vi "avaliaBolaDentroArea.vi"(10 "balls":T1[](array[typedef]), 11 "IA State":T2={"our_robots"=[], "enemy_robots"=[], "balls"=[], "geometry"={"field_length"=0, "field_width"=0, "goal_width"=0, "goal_depth"=0, "center_circle_radius"=0, "defense_width"=0, "defense_depth"=0, "free_kick_from_defense_dist"=0, "penalty_spot_from_field_line_dist"=0, "penalty_line_from_spot_dist"=0, "half_moon_depth"=0, "half_moon_width"=0}, "IA Judge"={"stage"="", "command"="", "our_goalie_id"=0.0, "enemy_goalie_id"=0.0, "command enum"=enum."Halt", "Time"=enum."Azul"}, "Received Timestamp"=timestamp(0 s since 1904-01-01), "Events"={"Touch"=FALSE, "id touch"=0.0, "Ball out of \nVision"=FALSE, "Ball inside \nGoalie area"=FALSE, "Robot not responding"=FALSE, "Robots responding status"=[1.0, 1.0, 1.0, 1.0, 1.0, 1.0], "Enemy Ball \nPossession"=FALSE, "Id ini Possession"=0.0, "Ball Possesion"=FALSE, "Id Possesion"=0.0, "Ball at\nour goal side"=FALSE, "Ball at\ntouchline"=FALSE, "Ball at\nenemy goal side"=FALSE}}) -> (3 "Bola dentro da área":bool=TRUE)   [LabVIEW 2018]
uses:
  2019/VSS/Core/AI Input.ctl
  2019/VSS/Core/AI Robot.ctl
  2019/VSS/Intel/Functions Enum.ctl
  2019/VSS/Intel/AttackerStates.ctl
  2019/VSS/Path Planning/RRT/PathDests.ctl
  2019/VSS/Path Planning/RRT/PathDest.ctl
  2019/VSS/Core/AI Ball.ctl
  2019/VSS/Core/Field Size.ctl
  2019/VSS/Core/AI Judge.ctl
  2019/VSS/Intel/Command Enum.ctl
  2019/VSS/Util/Events/Events.ctl
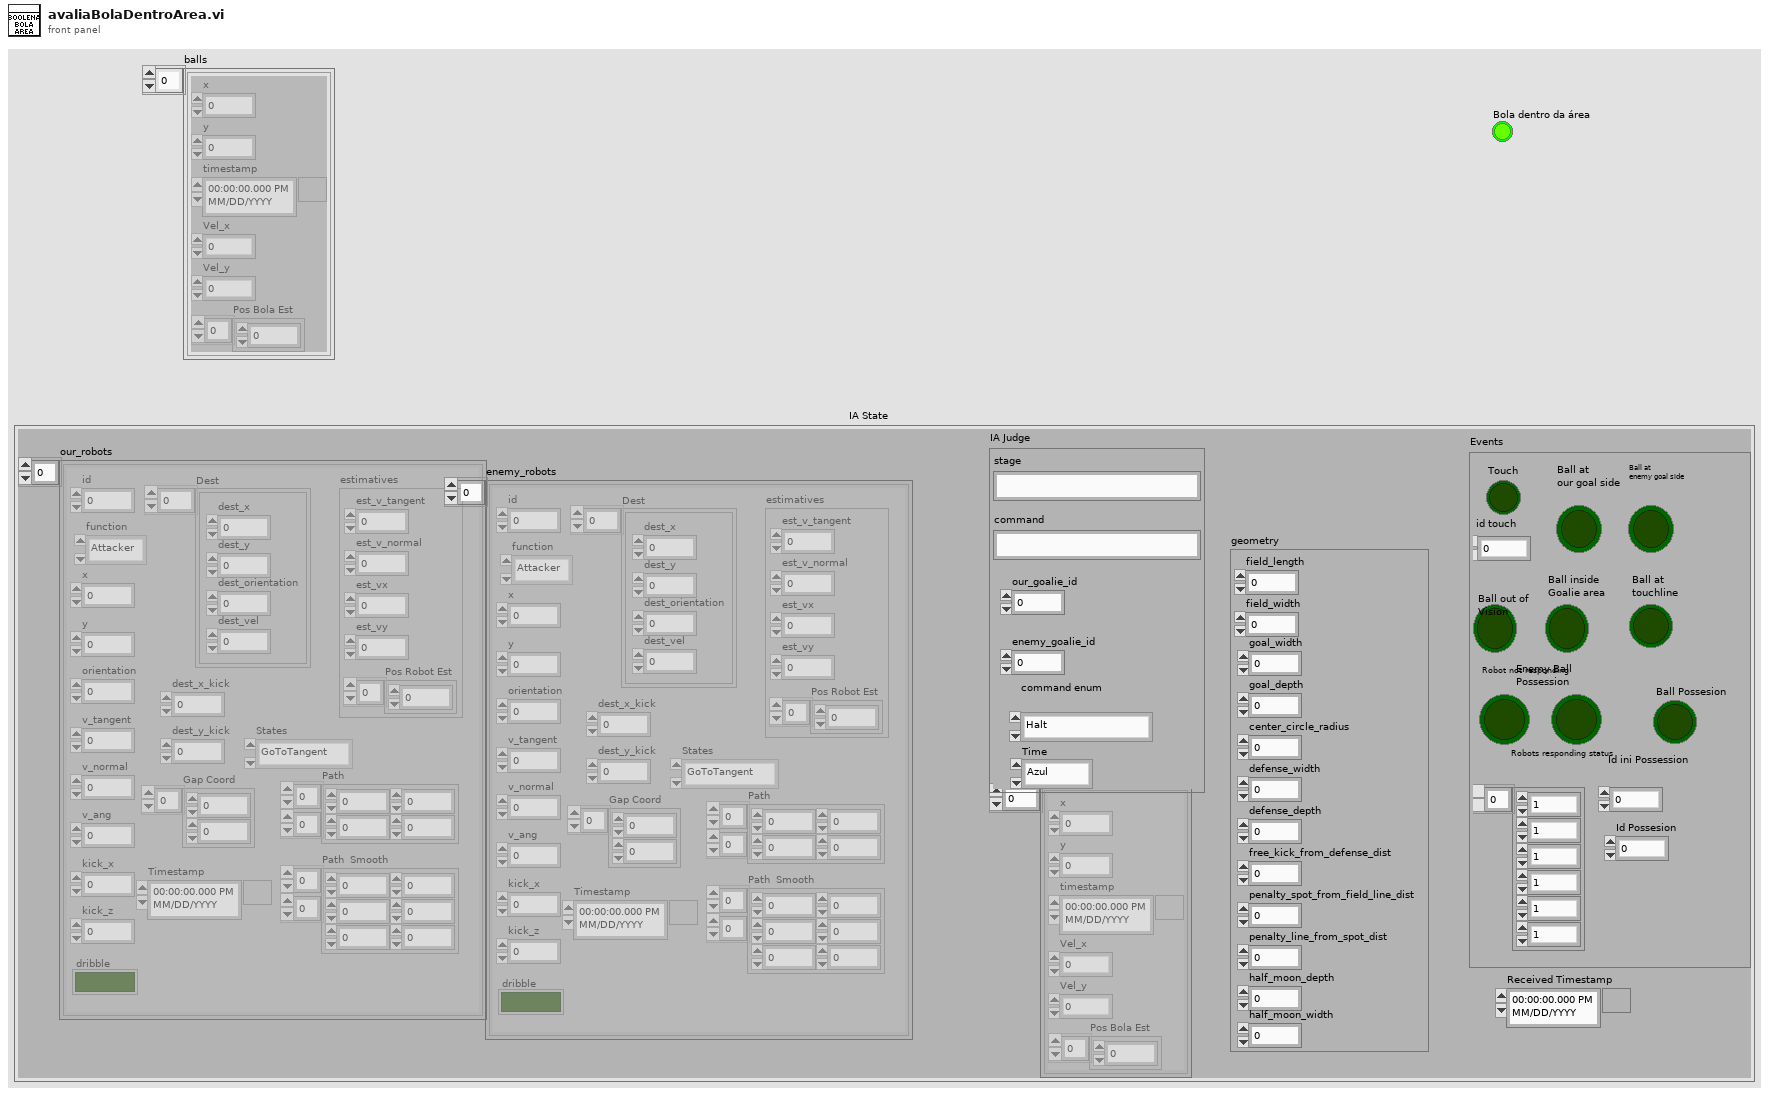
[diagram p1: front panel]
types:
  T1 = typedef "AI Ball.ctl" = cluster{"x":dbl, "y":dbl, "timestamp":timestamp, "Vel_x":dbl, "Vel_y":dbl, "Pos Bola Est":dbl[]}
  T2 = typedef "AI Input.ctl" = cluster{"our_robots":T3[], "enemy_robots":T3[], "balls":T1[], "geometry":T8, "IA Judge":T9, "Received Timestamp":timestamp, "Events":T11}
  T3 = typedef "AI Robot.ctl" = cluster{"id":u32, "function":T4, "x":dbl, "y":dbl, "orientation":dbl, "v_tangent":dbl, "v_normal":dbl, "v_ang":dbl, "kick_x":dbl, "kick_z":dbl, "dribble":bool, "Timestamp":timestamp, "estimatives":cluster{"est_v_tangent":dbl, "est_v_normal":dbl, "est_vx":dbl, "est_vy":dbl, "Pos Robot Est":dbl[]}, "dest_x_kick":dbl, "dest_y_kick":dbl, "Gap Coord":dbl[], "States":T5, "Path ":dbl[][], "Path  Smooth":dbl[][], "Dest":T6}
  T4 = typedef "Functions Enum.ctl" = enum16{"Attacker", "Goalie", "Defender", "Striker", "Goto 0", "Dummy", "Kicker", "ZigZag"}
  T5 = typedef "AttackerStates.ctl" = enum16{"Pass", "GoToTangent", "BallGetting", "GoToKick", "Rotate anti-clockwise", "Rotate Clockwise", ""}
  T6 = typedef "PathDests.ctl" = T7[]
  T7 = typedef "PathDest.ctl" = cluster{"dest_x":dbl, "dest_y":dbl, "dest_orientation":dbl, "dest_vel":dbl}
  T8 = typedef "Field Size.ctl" = cluster{"field_length":u32, "field_width":u32, "goal_width":u32, "goal_depth":u32, "center_circle_radius":u32, "defense_width":u32, "defense_depth":u32, "free_kick_from_defense_dist":u32, "penalty_spot_from_field_line_dist":u32, "penalty_line_from_spot_dist":u32, "half_moon_depth":u32, "half_moon_width":u32}
  T9 = typedef "AI Judge.ctl" = cluster{"stage":string, "command":string, "our_goalie_id":dbl, "enemy_goalie_id":dbl, "command enum":T10, "Time":enum16{"Azul", "Amarelo"}}
  T10 = typedef "Command Enum.ctl" = enum16{"Halt", "Stop", "Force Start", "PKA Normal Start", "Prepare Kickoff Ally", "PKE Normal Start", "Prepare Kickoff Enemy", "Prepare Penalty Ally", "PPA Normal Start", "Prepare Penalty Enemy", "PPE Normal Start", "Ball Placement Enemy Up", "Ball Placement Enemy Down", "Ball Placement Ally Up", "Ball Placement Ally Mid", "Ball Placement Ally Down", "Indirect Free Enemy", "Indirect Free Ally", "Timeout Enemy", "Timeout Ally", "Goal Enemy", "Goal Ally", "Normal Half Time", "Extra Time Break", "Extra Half Time", "None", "Post Game"}
  T11 = typedef "Events.ctl" = cluster{"Touch":bool, "id touch":dbl, "Ball out of \nVision":bool, "Ball inside \nGoalie area":bool, "Robot not responding":bool, "Robots responding status":dbl[], "Enemy Ball \nPossession":bool, "Id ini Possession":dbl, "Ball Possesion":bool, "Id Possesion":dbl, "Ball at\nour goal side":bool, "Ball at\ntouchline":bool, "Ball at\nenemy goal side":bool}
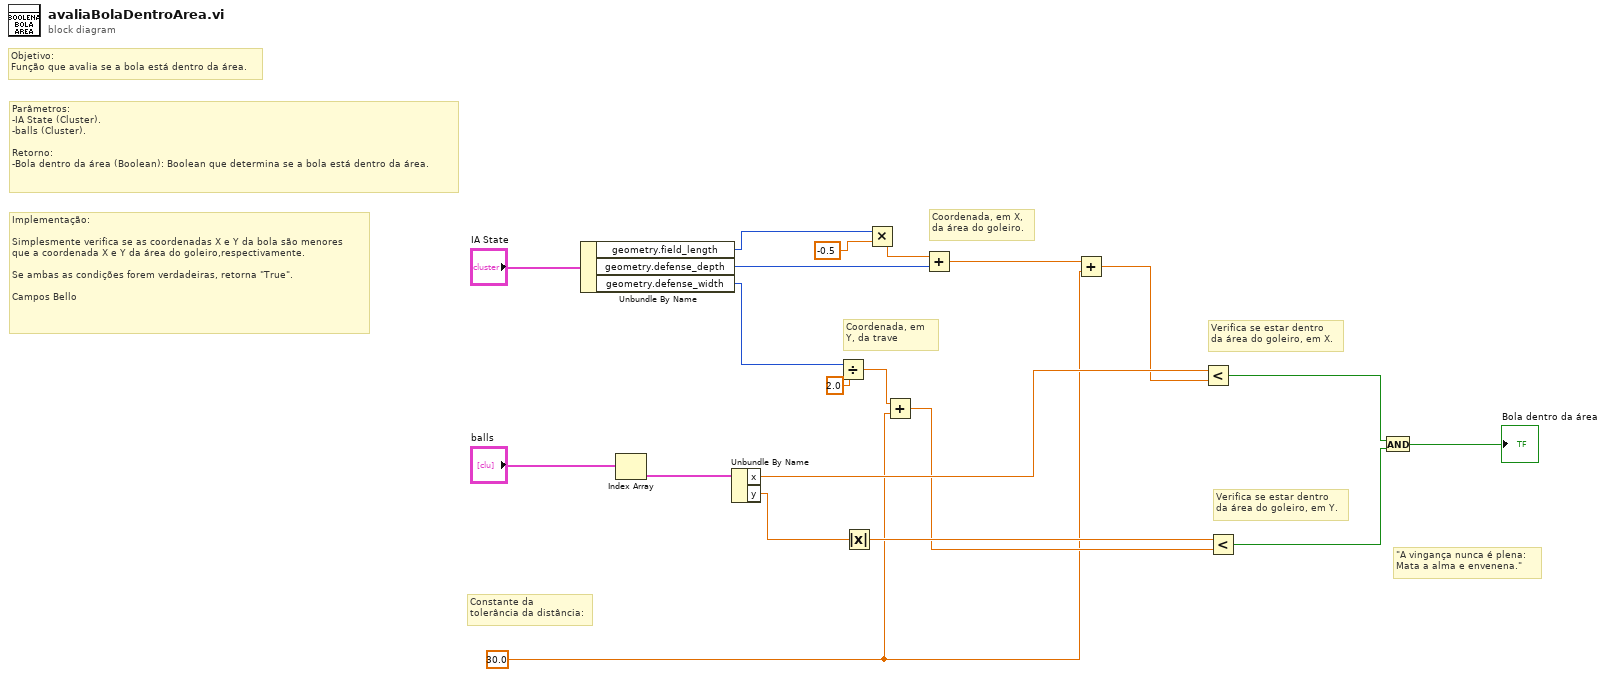
[diagram p0: block diagram]
diagram:
  w1 = 30.0
  # "Constante da\ntolerância da distância:"
  # "\"A vingança nunca é plena:\nMata a alma e envenena.\""
  # "Implementação:\n\nSimplesmente verifica se as coordenadas X e Y da bola são menores\nque a coordenada X e Y da área do goleiro,respectivamente.\n\nSe ambas as condições forem verdadeiras, retorna \"True\".\n\nCampos Bello"
  # "Parâmetros:\n-IA State (Cluster).\n-balls (Cluster).\n\nRetorno:\n-Bola dentro da área (Boolean): Boolean que determina se a bola está dentro da área."
  # "Objetivo:\nFunção que avalia se a bola está dentro da área."
  # "Verifica se estar dentro\nda área do goleiro, em Y."
  # "Verifica se estar dentro\nda área do goleiro, em X."
  # "Coordenada, em X,\nda área do goleiro."
  # "Coordenada, em \nY, da trave"
  n1 = Unbundle By Name("IA State") -> ("geometry.field_length"=w16:u32, "geometry.defense_depth"=w15:u32, "geometry.defense_width"=w11:u32)
  n2 = Index Array(array="balls") -> (element=w19:T1)  [unwired: 1 in]
  n3 = Unbundle By Name(w19) -> ("x"=w13:dbl, "y"=w10:dbl)
  n4 = Divide(x=w11, y=2.0 ("x/y")) -> (x/y=w3:dbl)
  n5 = Absolute Value(x=w10) -> (abs(x)=w9:dbl)
  n6 = Multiply(x=w16, y=-0.5) -> (x*y=w14:dbl)
  n7 = Add(x=w3, y=w1) -> (x+y=w2:dbl)
  n8 = Add(x=w14, y=w15) -> (x+y=w5:dbl)
  n9 = Add(x=w5, y=w1) -> (x+y=w4:dbl)
  n10 = Less?(x=w13, y=w4) -> (x < y?=w8:bool)
  n11 = Less?(x=w9, y=w2) -> (x < y?=w7:bool)
  n12 = And(x=w8, y=w7) -> (x .and. y?=→"Bola dentro da área":bool)
